vi "transform_point.vi"(10 "transformation parameters":T1={"1/Zoom"=1.0, "sin Phi"=0.0, "cos Phi"=1.0} {"cos Phi" format="%.35g"; "sin Phi" format="%.35g"; "1/Zoom" format="%.35g"}, 11 "scan point in":T2) -> (3 "scan point out":T2)   [LabVIEW 2010]
uses:
  scan_point_cluster.ctl
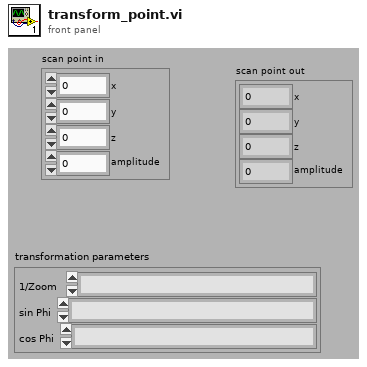
[diagram p1: front panel]
types:
  T1 = cluster{"1/Zoom":fxp<+,36,2>, "sin Phi":fxp<+/-,36,2>, "cos Phi":fxp<+/-,36,2>}
  T2 = typedef "scan_point_cluster.ctl" = cluster{"x":u16, "y":u16, "z":u16, "amplitude":u16}
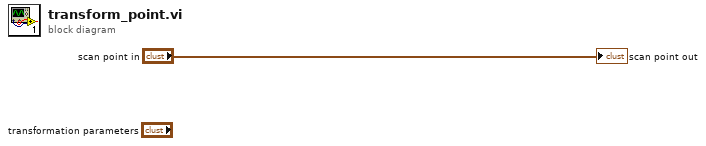
[diagram p0: block diagram]
diagram:
  "scan point out" <- "scan point in"
